vi "CS_LFAClassGlobal.vi"() -> ()   [LabVIEW 2013, in "LightField Automation.lvclass"]
uses:
  LightField Automation.lvclass
panel:
  in  "LightField Automation.lvclass":refnum<class "LightField Automation.lvclass">
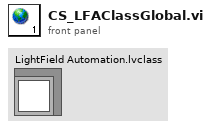
[diagram p1: front panel]
diagram:
